vi "thermal_optical_camera_V1.vi"() -> ()   [LabVIEW 2025]
uses:
  <vilib>/vision/driver/NI_Vision_Acquisition_Software.lvlib
panel:
  in  "File Path":string="C:\\Digambar\\Metal_thin_wall\\Optical_images\\Optical_images"
  in  "Stop (F)":bool
  in  "Acquisition Control:\nExposure Time [100, 3E7]":dbl=999.0 caption="Acquisition Control::Exposure Time" min=100.0 max=29999995.0
  in  "Analog Control:\nGain [0, 27]":dbl caption="Analog Control::Gain" min=0.0 max=27.045663671679687
  in  "Analog Control:\nBlack Level [-5, 10]":dbl caption="Analog Control::Black Level" min=-5.0000011920928955 max=10.000002384185791
  in  "Analog Control:\nGamma [0.25, 4.00]":dbl=0.800048828125 caption="Analog Control::Gamma" min=0.25 max=4.0 step=0.05
  out "Frames":i32
  out "Optical camera":T1(plugin-control)
  in  "capture interval (s) for optical camera":dbl
  out "Camera Information Array":T2(array[cluster]) {"BusType" format="%x"; "SerialNumberLow" format="%.0x"; "SerialNumberHigh" format="%.0x"}
  in  "Connected Only? (Yes)":bool=TRUE
  in  "capture interval (s) for thermal camera":dbl
  out "Thermal camera":T1(plugin-control)
  out "IP address":string
  out "Output":string
  in  "Flag":bool
  in  "Stop recording":bool
  in  "Stop Preview":bool
  in  "Focus":dbl(slide) scale=0.0..100.0
  in  "Record":bool
  out "?":string
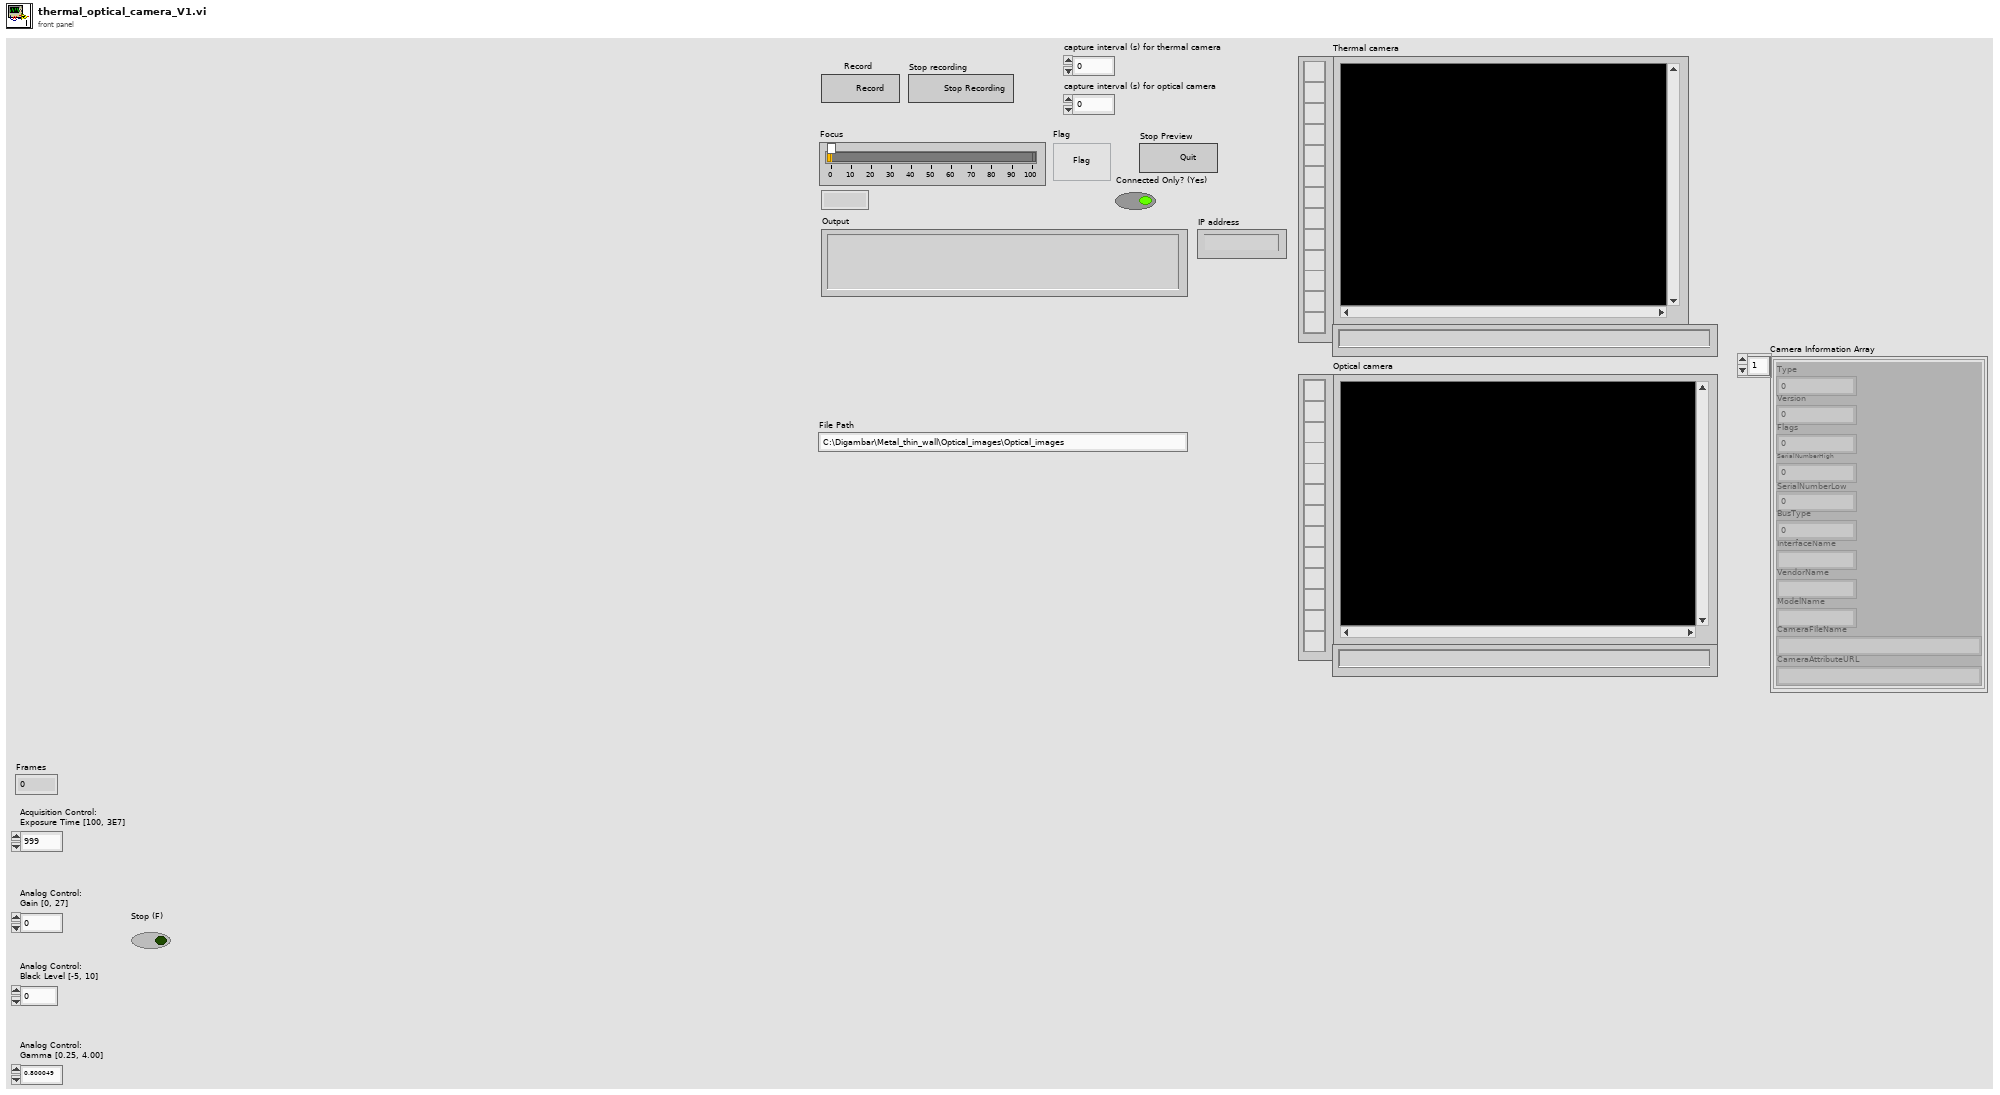
[diagram p1: front panel]
types:
  T1 = typedef "IMAQ Image.ctl" = refnum<image>
  T2 = cluster{"Type":u32, "Version":u32, "Flags":u32, "SerialNumberHigh":u32, "SerialNumberLow":u32, "BusType":u32, "InterfaceName":string, "VendorName":string, "ModelName":string, "CameraFileName":string, "CameraAttributeURL":string}[]
  T3 = enum16{"open", "replace", "create", "open or create", "replace or create", "replace or create with confirmation"}
  T4 = enum16{"big-endian, network order", "native, host order", "little-endian"}
  T5 = enum16{"Standard", "Buffered", "CRLF", "Immediate"}
  T6 = typedef "Image Type" = u32
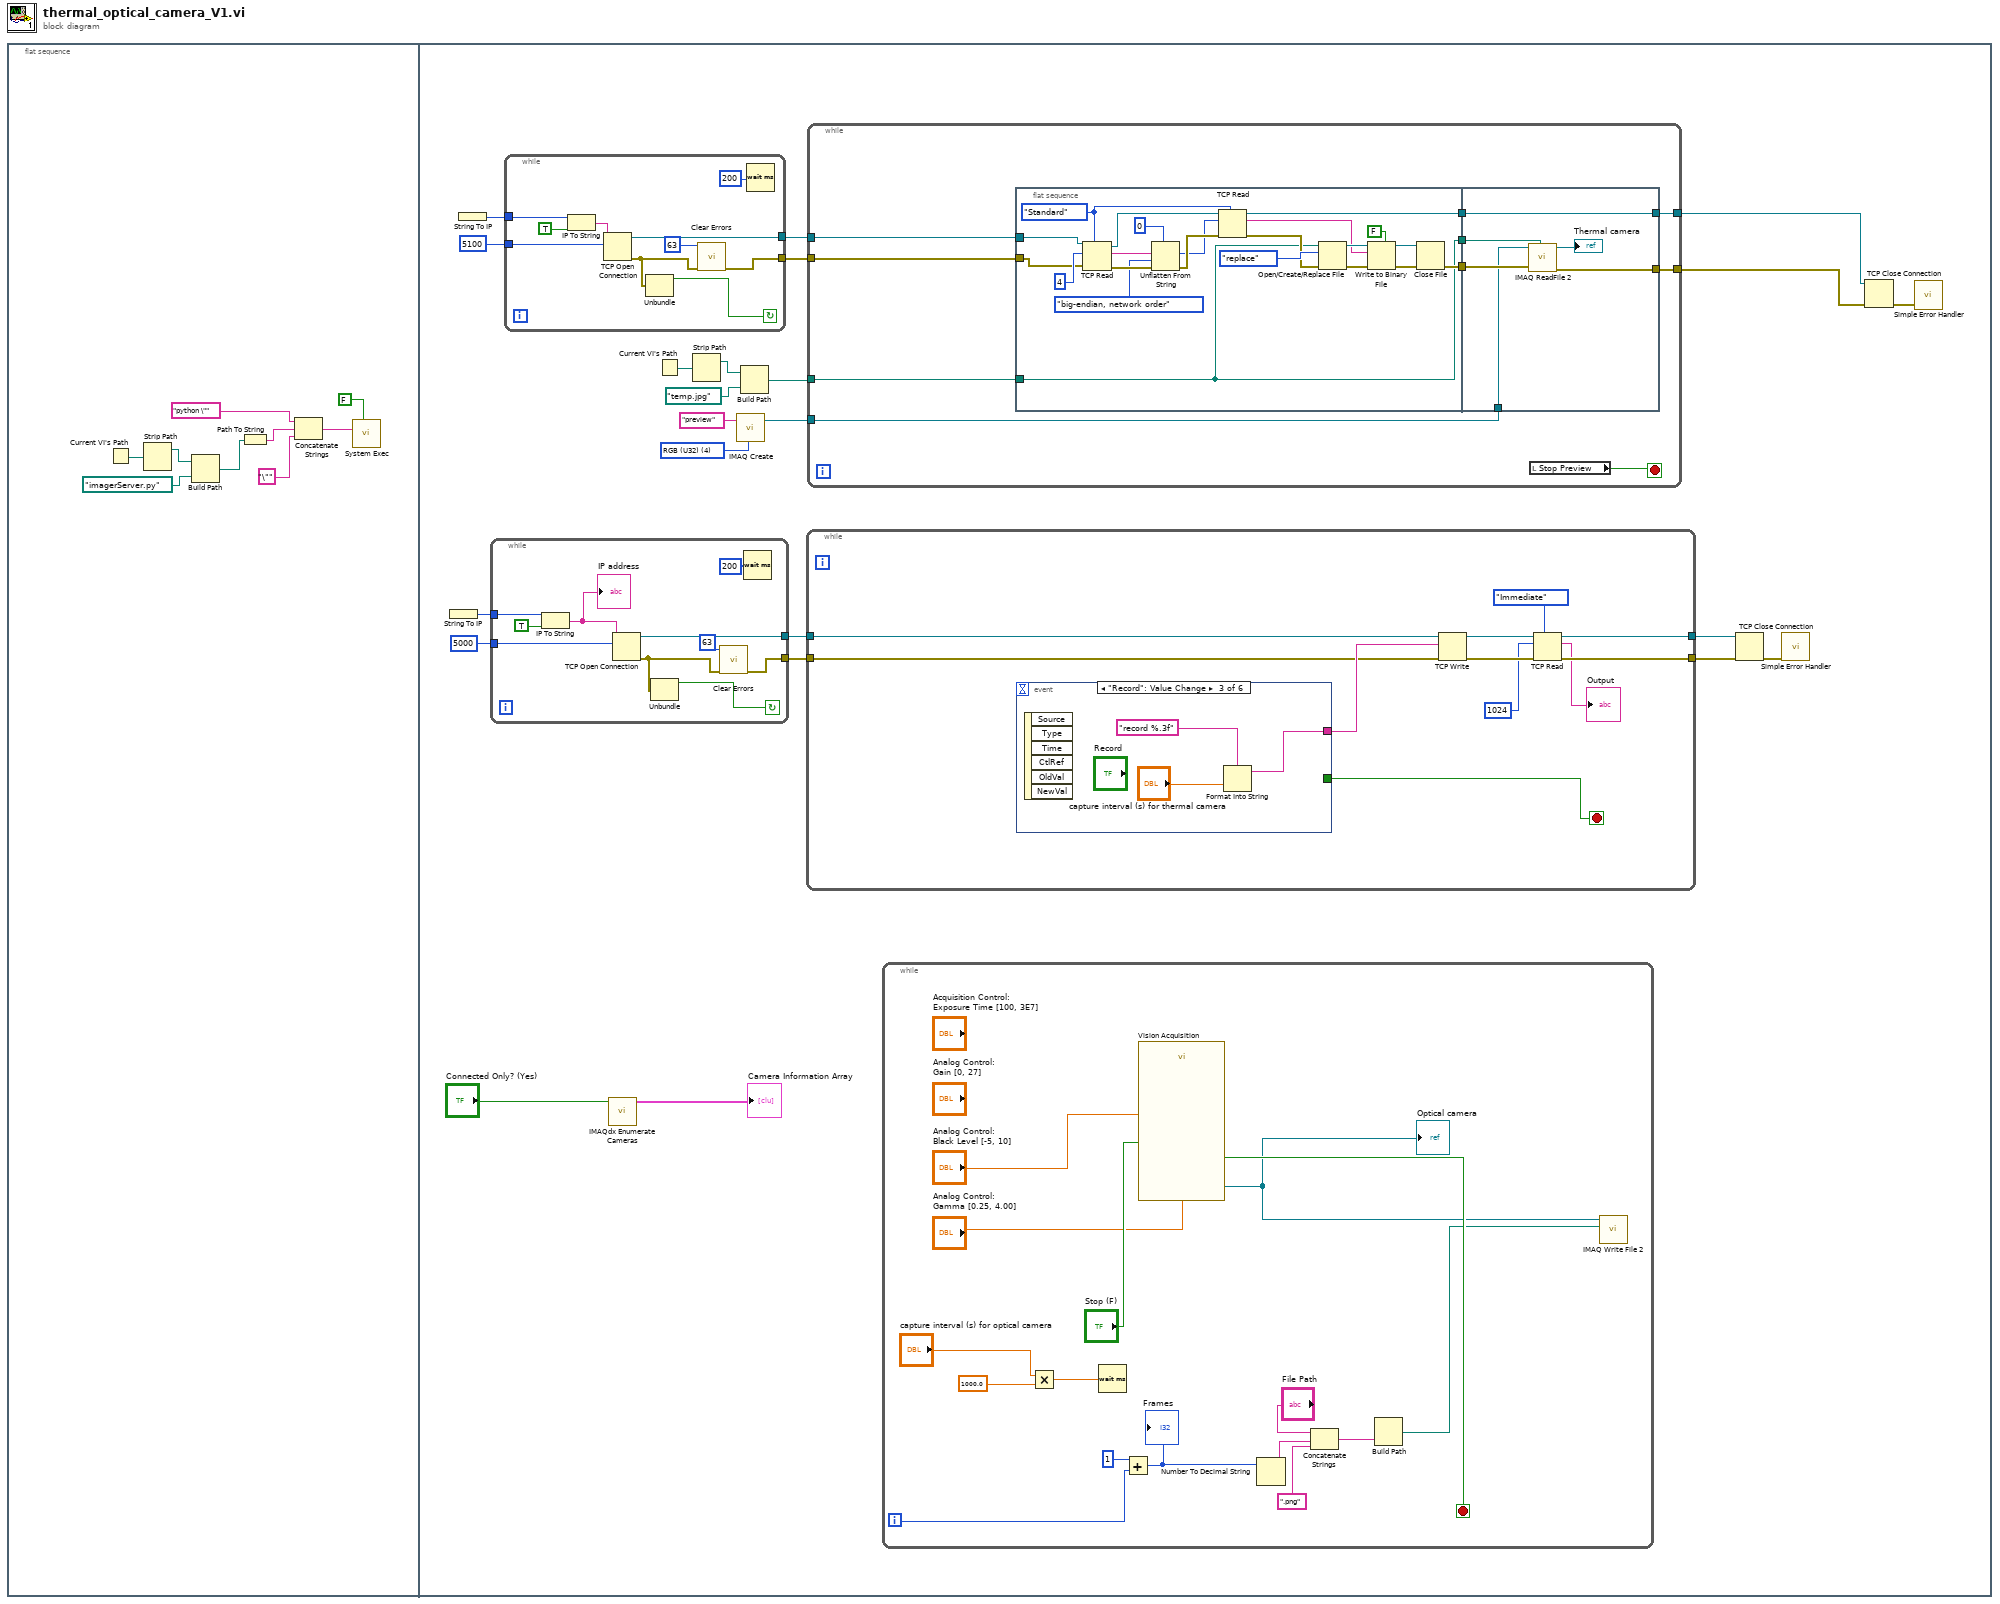
[diagram p0: block diagram]
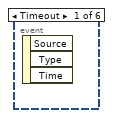
[diagram p2: hidden frame]
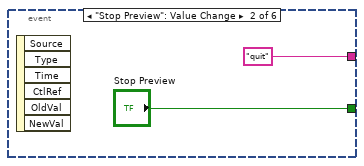
[diagram p3: hidden frame]
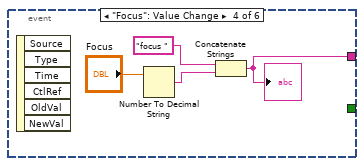
[diagram p4: hidden frame]
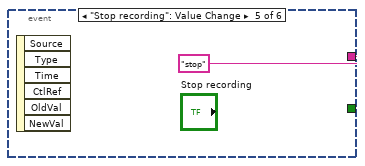
[diagram p5: hidden frame]
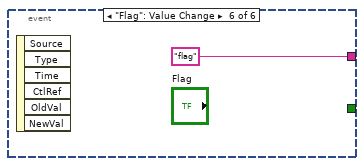
[diagram p6: hidden frame]
diagram:
  n1 = flat-sequence {
    frame #0 {
      n2 = Current VI's Path() -> (path=w4:path)
      n3 = Strip Path(path=w4) -> (stripped path=w5:path)  [unwired: 1 out]
      n4 = Build Path(base path=w5, name or relative path=path "imagerServer.py") -> (appended path=w2:path)
      n5 = Path To String(path=w2) -> (string=w8:string)
      n6 = Concatenate Strings("python \"" ("string"), w8, "\"" ("string")) -> (w7:string)
      n7 = call <vilib>:"System Exec.vi"("wait until completion? (T)"=FALSE, "command line"=w7) -> ()  [unwired: 6 in, 4 out]
    }
    frame #1 {
      w20 = T6 4 items=["Grayscale (U8)", "Grayscale (I16)", "Grayscale (SGL)", "Complex (CSG)", "RGB (U32)", "HSL (U32)", "RGB (U64)", "Grayscale (U16)"] ("Image Type")
      n8 = String To IP() -> (0:w17:u32)  [unwired: 1 in]
      n9 = String To IP() -> (0:w15:u32)  [unwired: 1 in]
      n10 = while {
        tunnel: [w62] -> w19
        tunnel: [w68] -> w18
        tunnel: w17 -> [w66]
        tunnel: u16 5000 ("remote port or service name") -> [w64]
        stop <- w59 continue-if-true
        n11 = IP To String(1:TRUE ("dot notation? (F)"), 2:w66) -> (0:w67:string)
        "IP address" <- w67
        n12 = TCP Open Connection(address=w67, remote port or service name=w64) -> (connection ID=w68:refnum<k5>, error out=w63:errorcluster)  [unwired: 3 in]
        n13 = Unbundle(w63) -> ("status"=w59:bool)  [unwired: 2 out]
        n14 = call <vilib>:"Clear Errors.vi"("error in (no error)"=w63, "specific error code to clear (0: all)"=63) -> ("error out"=w62:errorcluster)  [unwired: 4 in, 1 out]
        n15 = Wait (ms)(milliseconds to wait=u32 200) -> ()  [unwired: 1 out]
      }
      n16 = while {
        tunnel: w15 -> [w58]
        tunnel: [w52] -> w14
        tunnel: [w56] -> w13
        tunnel: u16 5100 ("remote port or service name") -> [w54]
        stop <- w49 continue-if-true
        n17 = IP To String(1:TRUE ("dot notation? (F)"), 2:w58) -> (0:w57:string)
        n18 = TCP Open Connection(address=w57, remote port or service name=w54) -> (connection ID=w56:refnum<k5>, error out=w53:errorcluster)  [unwired: 3 in]
        n19 = Unbundle(w53) -> ("status"=w49:bool)  [unwired: 2 out]
        n20 = call <vilib>:"Clear Errors.vi"("error in (no error)"=w53, "specific error code to clear (0: all)"=63) -> ("error out"=w52:errorcluster)  [unwired: 4 in, 1 out]
        n21 = Wait (ms)(milliseconds to wait=u32 200) -> ()  [unwired: 1 out]
      }
      n22 = call <vilib>:"IMAQdx Enumerate Cameras.vi"("Connected Only? (Yes)"="Connected Only? (Yes)") -> ("Camera Information Array"=→"Camera Information Array":T2)  [unwired: 9 in, 1 out]
      n23 = Current VI's Path() -> (path=w31:path)
      n24 = Strip Path(path=w31) -> (stripped path=w32:path)  [unwired: 1 out]
      n25 = call "IMAQ Create"("Image Name"="preview", "Image Type"=w20) -> ("New Image"=w27:T1)  [unwired: 3 in, 1 out]
      n26 = Build Path(base path=w32, name or relative path=path "temp.jpg") -> (appended path=w30:path)
      n27 = while {
        tunnel: [w116] -> w23
        tunnel: [w114] -> w24
        tunnel: w19 -> [w112]
        tunnel: w18 -> [w111]
        stop <- w107 stop-if-true
        n28 = event shown="[2] \"Record\": Value Change" {
          selector: _ -> [_ _ _ _ _ _]
          dyn-events: _ -> [_ _ _ _ _ _]
          timeout: _ -> [_ _ _ _ _ _]
          tunnel: [_ "quit" w122 w124 "stop" "flag"] -> w113
          tunnel: [_ "Stop Preview" _ _ _ _] -> w107
          event Timeout {
            n29 = event-data() -> ()  [unwired: 1 in, 3 out]
          }
          event "Stop Preview": Value Change {
            n30 = event-data() -> ()  [unwired: 1 in, 6 out]
          }
          event "Record": Value Change {
            n31 = event-data() -> ()  [unwired: 1 in, 6 out]
            n32 = Format Into String(format string="record %.3f", "capture interval (s) for thermal camera") -> (resulting string=w122:string)  [unwired: 2 in, 1 out]
          }
          event "Focus": Value Change {
            n33 = event-data() -> ()  [unwired: 1 in, 6 out]
            n34 = Number To Decimal String(number="Focus") -> (decimal integer string=w126:string)  [unwired: 1 in]
            n35 = Concatenate Strings("focus ", w126) -> (w124:string)
            "?" <- w124
          }
          event "Stop recording": Value Change {
            n36 = event-data() -> ()  [unwired: 1 in, 6 out]
          }
          event "Flag": Value Change {
            n37 = event-data() -> ()  [unwired: 1 in, 6 out]
          }
        }
        n38 = TCP Write(connection ID=w111, data in=w113, error in (no error)=w112) -> (connection ID out=w115:refnum<k5>, error out=w117:errorcluster)  [unwired: 1 in, 1 out]
        n39 = TCP Read(connection ID=w115, bytes to read=1024, error in (no error)=w117, 7:T5."Immediate" ("mode (standard)")) -> (connection ID out=w114:refnum<k5>, data out=→"Output":string, error out=w116:errorcluster)  [unwired: 1 in]
      }
      n40 = while {
        tunnel: w27 -> [w73]
        tunnel: [w74] -> w28
        tunnel: [w78] -> w29
        tunnel: w30 -> [w76]
        tunnel: w14 -> [w71]
        tunnel: w13 -> [w70]
        stop <- w69 stop-if-true
        n41 = flat-sequence {
          tunnel: w76 -> [w82]
          tunnel: [w84] -> w77
          tunnel: [w83] -> w75
          tunnel: [w82] -> w72
          tunnel: w71 -> [w80]
          tunnel: w70 -> [w79]
          tunnel: [w106] -> w78
          tunnel: w77 -> [w106]
          tunnel: w75 -> [w105]
          tunnel: [w104] -> w74
          tunnel: w73 -> [w103]
          tunnel: w72 -> [w102]
          frame #0 {
            w93 = T5."Standard" ("mode (standard)")
            n42 = TCP Read(connection ID=w79, bytes to read=4, error in (no error)=w80, 7:w93) -> (connection ID out=w96:refnum<k5>, data out=w81:string, error out=w99:errorcluster)  [unwired: 1 in]
            n43 = Unflatten From String(type=0, binary string=w81, byte order (0:big-endian, network order)=T4."big-endian, network order", error in (no error)=w99) -> (value=w94:i32, error out=w95:errorcluster)  [unwired: 1 in, 1 out]
            n44 = TCP Read(connection ID=w96, bytes to read=w94, error in (no error)=w95, 7:w93) -> (connection ID out=w84:refnum<k5>, data out=w89:string, error out=w91:errorcluster)  [unwired: 1 in]
            n45 = Open/Create/Replace File(file path (use dialog)=w82, error in=w91, operation (0:open)=T3."replace") -> (refnum out=w90:refnum<file>, error out=w87:errorcluster)  [unwired: 3 in, 1 out]
            n46 = Write to Binary File(file (use dialog)=w90, data=w89, error in=w87, 5:FALSE ("prepend array or string size? (T)")) -> (refnum out=w85:refnum<file>, error out=w86:errorcluster)  [unwired: 2 in, 1 out]
            n47 = Close File(refnum=w85, error in=w86) -> (error out=w83:errorcluster)  [unwired: 1 out]
          }
          frame #1 {
            n48 = call "IMAQ ReadFile 2"("File Path"=w102, "error in (no error)"=w105, "Image"=w103) -> ("error out"=w104:errorcluster, "Image Out"=→"Thermal camera":T1)  [unwired: 4 in, 3 out]
          }
        }
        n49 = local read "Stop Preview"() -> (w69:bool)
      }
      n50 = while {
        i -> [w35]
        stop <- w47 stop-if-true
        n51 = Multiply(x="capture interval (s) for optical camera", y=1000.0) -> (x*y=w37:dbl)
        n52 = Wait (ms)(milliseconds to wait=w37) -> ()  [unwired: 1 out]
        n53 = Add(x=1, y=w35) -> (x+y=w43:i32)
        "Frames" <- w43
        n54 = call "Vision Acquisition"("Analog Control::Black Level"="Analog Control:\nBlack Level [-5, 10]", "Analog Control::Gamma"="Analog Control:\nGamma [0.25, 4.00]", "Stop (F)"="Stop (F)") -> ("Image Out"=w46:T1, "Stopped"=w47:bool)  [unwired: 22 in, 1 out]
        "Optical camera" <- w46
        n55 = Number To Decimal String(number=w43) -> (decimal integer string=w38:string)  [unwired: 1 in]
        n56 = Concatenate Strings("File Path", w38, ".png" ("string")) -> (w41:string)
        n57 = Build Path(name or relative path=w41) -> (appended path=w34:path)  [unwired: 1 in]
        n58 = call-poly "IMAQ Write File 2"("File Path"=w34, "Image"=w46) -> ()  [unwired: 8 in, 2 out]
      }
      n59 = TCP Close Connection(connection ID=w24, error in (no error)=w23) -> (error out=w25:errorcluster)  [unwired: 1 in, 1 out]
      n60 = call <vilib>:"Simple Error Handler.vi"("error in (no error)"=w25) -> ()  [unwired: 4 in, 5 out]
      n61 = TCP Close Connection(connection ID=w29, error in (no error)=w28) -> (error out=w26:errorcluster)  [unwired: 1 in, 1 out]
      n62 = call <vilib>:"Simple Error Handler.vi"("error in (no error)"=w26) -> ()  [unwired: 4 in, 5 out]
    }
  }
